vi "ReadFileWRONG.vi"(10 "Location":string) -> (2 "Array - Numeric":dbl[][](array[numeric]))   [LabVIEW 2016]
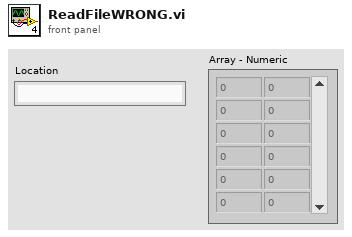
[diagram p1: front panel]
types:
  T1 = enum16{"open", "replace", "create", "open or create", "replace or create", "replace or create with confirmation"}
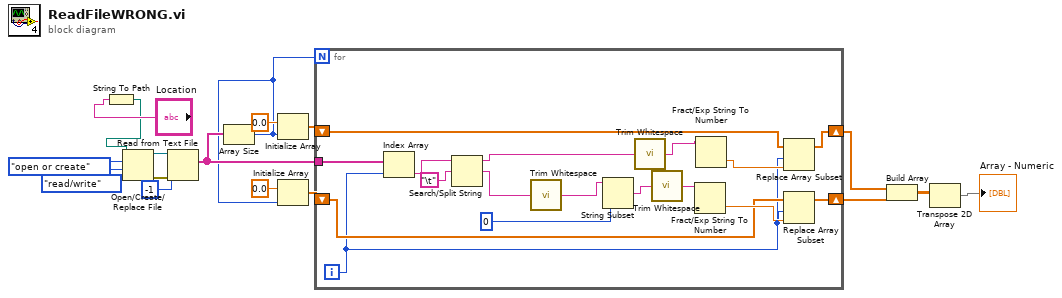
[diagram p0: block diagram]
diagram:
  n1 = String To Path(string="Location") -> (path=w1:path)
  n2 = Open/Create/Replace File(file path (use dialog)=w1, operation (0:open)=T1."open or create", access (0:read/write)=enum16{"read/write", "read-only", "write-only"}."read/write") -> (refnum out=w15:refnum<file>, error out=w14:errorcluster)  [unwired: 3 in, 1 out]
  n3 = Read from Text File(file (use dialog)=w15, count=-1, error in=w14) -> (text=w12:string[])  [unwired: 1 in, 3 out]
  n4 = Array Size(array=w12) -> (size(s)=w9:i32)
  n5 = Initialize Array(0.0 ("element"), w9) -> (w10:dbl[])
  n6 = Initialize Array(0.0 ("element"), w9) -> (w7:dbl[])
  n7 = for {
    N: w9 -> [_]
    tunnel: w12 -> [w28]
    shift-right: [w22] -> w6
    shift-left: w10 -> [w27]
    shift-right: [w21] -> w5
    shift-left: w7 -> [w24]
    i -> [w23]
    n8 = Index Array(array=w28, index=w23) -> (element=w34:string)
    n9 = Search/Split String(string=w34, search string/char (-)="\t") -> (substring before match=w33:string, match + rest of string=w20:string)  [unwired: 1 in, 1 out]
    n10 = call <vilib>:"Trim Whitespace.vi"("string"=w20) -> ("trimmed string"=w19:string)  [unwired: 1 in]
    n11 = String Subset(string=w19, offset (0)=0) -> (substring=w32:string)  [unwired: 1 in]
    n12 = call <vilib>:"Trim Whitespace.vi"("string"=w33) -> ("trimmed string"=w30:string)  [unwired: 1 in]
    n13 = call <vilib>:"Trim Whitespace.vi"("string"=w32) -> ("trimmed string"=w29:string)  [unwired: 1 in]
    n14 = Fract/Exp String To Number(string=w29) -> (number=w25:dbl)  [unwired: 3 in, 1 out]
    n15 = Fract/Exp String To Number(string=w30) -> (number=w26:dbl)  [unwired: 3 in, 1 out]
    n16 = Replace Array Subset(array=w27, new element=w26, index=w23) -> (w22:dbl[])
    n17 = Replace Array Subset(array=w24, new element=w25, index=w23) -> (w21:dbl[])
  }
  n18 = Build Array(w6, w5) -> (w4:dbl[][])
  n19 = Transpose 2D Array(2D array=w4) -> (transposed array=→"Array - Numeric":dbl[][])
